vi "Modem Status specific Variable List.vi"(11 "error in (no error)":errorcluster) -> (15 "error out":errorcluster)   [LabVIEW 2011]
uses:
  emi Lib/Basic/0 - General/App/emi_Application Folder.vi
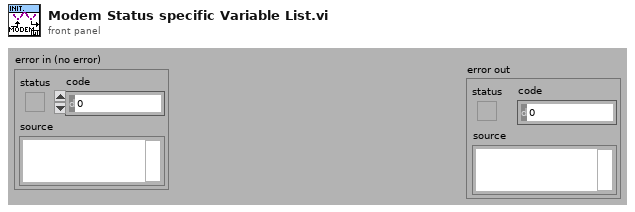
[diagram p1: front panel]
types:
  T1 = typedef "Fixed Analog Channel Definition.ctl" = cluster{"ID":u16, "Name":string, "Quantity":T2, "Unit":string, "Maximum upd":T3, "Comment":string, "Help file Name":string, "Help file Section ":string, "Category":T4, "User adjustable Scaling":bool, "Default Scaling":T5, "Default Unit":i32, "Classification":T6}
  T2 = typedef "Quantity enum.ctl" = enum16{"NA", "Acceleration", "Angle", "Current", "Force", "Distance", "Pressure", "Resistance", "Rotational Speed", "Speed", "Temperature", "Tension", "Torque", "Voltage", "Weight"}
  T3 = typedef "Update frequensies.ctl" = enum16{"2 Hz", "1 Hz", "0.1 Hz"}
  T4 = typedef "Channel catagory Enum.ctl" = enum16{"No Category", "Power", "Temperature", "Pressure"}
  T5 = typedef "Scaling.ctl" = cluster{"Gain":dbl, "Offset":dbl}
  T6 = typedef "Channel Classification Enum.ctl" = enum16{"Basic", "Advanced", "Expert", "Unused"}
  T7 = typedef "Fixed Digital Channel Definition.ctl" = cluster{"ID":u16, "Name":string, "NA Text":string, "Off Text":string, "On Text":string, "Maximum upd":T3, "Comment":string, "Help file Name":string, "Help file Section ":string, "Catagory":T4, "In use":bool}
  T8 = typedef "User Setting DigitalChannel.ctl" = cluster{"Responses":cluster{"Technical Error (NA)":T9, "OFF / FALSE":T11, "ON / TRUE":T11}}
  T9 = typedef "Alarm Responce.ctl" = cluster{"Action":T10, "Alarm":bool}
  T10 = typedef "Action List.ctl" = enum16{"No Action", "Stop Motor", "Turn Off HV"}
  T11 = typedef "Alarm Responce dig.ctl" = cluster{"Action":T10, "Alarm":bool, "Exclamation":bool}
  T12 = typedef "User Setting Analog Channel Bg.ctl" = cluster{"Scaling":T5, "Limits and responces":T13, "Allow Graph selection by user":bool, "Unit":u16}
  T13 = typedef "Alarm Setup Analog.ctl" = cluster{"Technical Error(NA)":T9, "LL":T9, "L":T9, "H":T9, "HH":T9, "Limits":T14}
  T14 = typedef "Limits.ctl" = cluster{"LL":dbl, "L":dbl, "H":dbl, "HH":dbl}
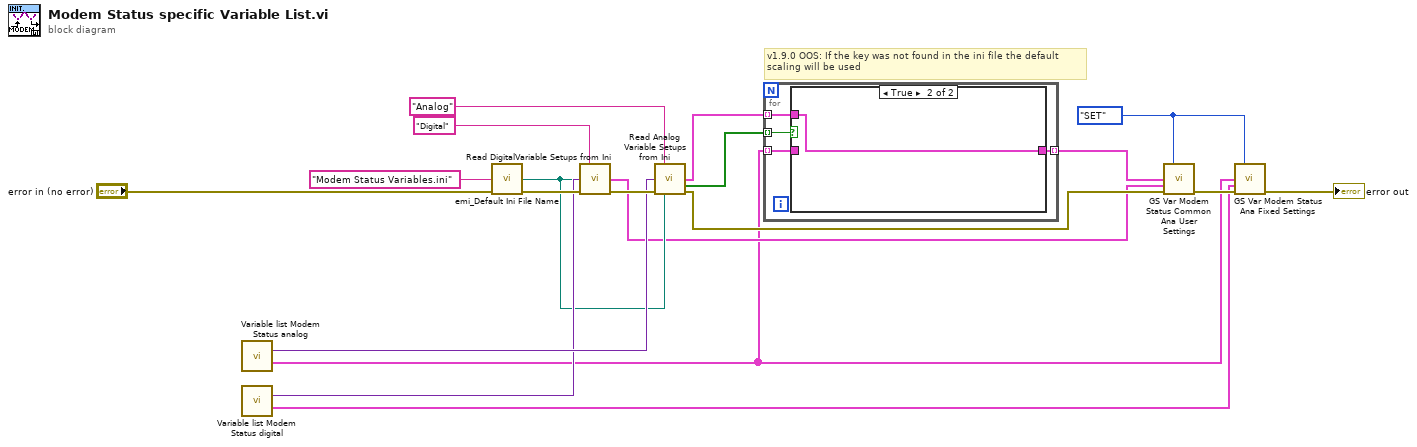
[diagram p0: block diagram]
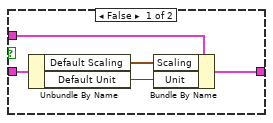
[diagram p2: hidden frame]
diagram:
  w1 = enum16{"GET", "SET"}."SET" ("Action(GET)")
  # "v1.9.0 OOS: If the key was not found in the ini file the default\nscaling will be used"
  n1 = call "Variable list Modem Status analog.vi"() -> ("Variant"=w14:variant, "Array"=w3:T1[])  [unwired: 14 in]
  n2 = call "Variable list Modem Status digital.vi"() -> ("Variant"=w11:variant, "Array"=w2:T7[])  [unwired: 14 in]
  n3 = call "emi_Default Ini File Name.vi"("Name"="Modem Status Variables.ini" ("name or relative path"), "error in (no error)"="error in (no error)") -> ("Path"=w10:path, "error out"=w13:errorcluster)  [unwired: 12 in]
  n4 = call "Read DigitalVariable Setups from Ini.vi"("error in (no error)"=w13, "Path"=w10, "Enum with Variable List"=w11, "Section(\"Default\")"="Digital" ("Section(\"Default\")")) -> ("error out"=w18:errorcluster, "Digitale User settigns"=w6:T8[])  [unwired: 10 in]
  n5 = call "Read Analog Variable Setups from Ini.vi"("error in (no error)"=w18, "Path"=w10, "Enum with Variable List"=w14, "Section(\"Default\")"="Analog" ("Section(\"Default\")")) -> ("error out"=w8:errorcluster, "Found out"=w15:bool[], "Analog User settigns"=w16:T12[])  [unwired: 9 in]
  n6 = for {
    tunnel: w16 -> [w22] mode=indexing
    tunnel: w15 -> [w23] mode=indexing
    tunnel: w3 -> [w21] mode=indexing
    tunnel: [w20] -> w7 mode=indexing
    n7 = case shown="True" w23 {
      tunnel: w22 -> [w28 w29]
      tunnel: w21 -> [w27 _]
      tunnel: [w24 w29] -> w20
      frame False {
        n8 = Unbundle By Name(w27) -> ("Default Scaling"=w26:T5, "Default Unit"=w25:i32)
        n9 = Bundle By Name(cluster=w28, "Scaling"=w26, "Unit"=w25) -> (w24:T12)
      }
      frame True {
      }
    }
  }
  n10 = call "GS Var Modem Status Common Ana User Settings.vi"("Action(GET)"=w1, "Modem Status analog var User settigns in"=w7, "Modem Status digital var User settigns in"=w6, "error in (no error)"=w8) -> ("error out"=w5:errorcluster)  [unwired: 9 in, 2 out]
  n11 = call "GS Var Modem Status Ana Fixed Settings.vi"("Action(GET)"=w1, "Modem Status Analog Var Fixed in"=w3, "Modem Status Digital Var Fixed in"=w2, "error in (no error)"=w5) -> ("error out"=→"error out":errorcluster)  [unwired: 9 in, 2 out]
